vi "Manuel Olcum ile Excele Atma.vi"() -> ()   [LabVIEW 2014]
panel:
  in  "ok":bool
  in  "Kelvin Yk-1":dbl format="%.5p"
  in  "Kelvin Yk":dbl format="%.5p"
  in  "Wagner Yk-1":dbl format="%.5p"
  in  "Wagner Yk":dbl format="%.5p"
  in  "1R Yk-1":dbl format="%.5p"
  in  "1R Yk":dbl format="%.5p"
  in  "10R Yk-1":dbl format="%.5p"
  in  "10R Yk":dbl format="%.5p"
  in  "Ana Denge Yk-1":dbl format="%.5p"
  in  "Ana Denge Yk":dbl format="%.5p"
  in  "Cp 1R":dbl format="%_1e"
  in  "Cp 10R":dbl format="%_1e"
  in  "Kelvin Y_2":dbl=2e-07 format="%_1e"
  in  "Kelivn Y_1":dbl=1e-06 format="%_1e"
  in  "Kelvin X_2":dbl=2e-07 format="%_1e"
  in  "Kelvin X_1":dbl=1e-06 format="%_1e"
  in  "Wagner Y_2":dbl=2e-05 format="%_1e"
  in  "Wagner Y_1":dbl=5e-05 format="%_1e"
  in  "Wagner X_2":dbl=2e-05 format="%_1e"
  in  "Wagner X_1":dbl=5e-05 format="%_1e"
  in  "1R Y_2":dbl=1e-05 format="%_1e"
  in  "1R Y_1":dbl=2e-05 format="%_1e"
  in  "1R X_2":dbl=1e-05 format="%_1e"
  in  "1R X_1":dbl=2e-05 format="%_1e"
  in  "10R Y_2":dbl=1e-05 format="%_1e"
  in  "10R Y_1":dbl=2e-05 format="%_1e"
  in  "10R X_2":dbl=1e-05 format="%_1e"
  in  "10R X_1":dbl=2e-05 format="%_1e"
  in  "AD Y_2":dbl=2e-07 format="%_1e"
  in  "AD Y_1":dbl=1e-06 format="%_1e"
  in  "AD X_2":dbl=2e-07 format="%_1e"
  in  "AD X_1":dbl=1e-06 format="%_1e"
  in  "Direnc 2":dbl format="%_1e"
  in  "Direnc 1":dbl format="%_1e"
  in  "Besleme":dbl=1.0
  in  "Frekans":dbl=1000.0
  in  "Kelvin Faz":dbl format="%.3p"
  in  "Wagner Faz":dbl format="%.3p"
  in  "1R Faz":dbl format="%.3p"
  in  "10R Faz":dbl format="%.3p"
  in  "Ana Denge Faz":dbl format="%.3p"
  in  "Kelvin Xk-1":dbl format="%.5p"
  in  "Kelvin Xk":dbl format="%.5p"
  in  "Wagner Xk-1":dbl format="%.5p"
  in  "Wagner Xk":dbl format="%.5p"
  in  "1R Xk-1":dbl format="%.5p"
  in  "1R Xk":dbl format="%.5p"
  in  "10R Xk-1":dbl format="%.5p"
  in  "10R Xk":dbl format="%.5p"
  in  "Ana Denge Xk-1":dbl format="%.5p"
  in  "Ana Denge Xk":dbl format="%.5p"
  # "Otomatik ölçüm alınabilmesi için gereken değerler"
  # "Ana Denge Ve Kelvin İçin Range Değeri"
  # "5uV"
  # "10R, 1R ve Wagner İçin Range Değeri"
  # "500uV"
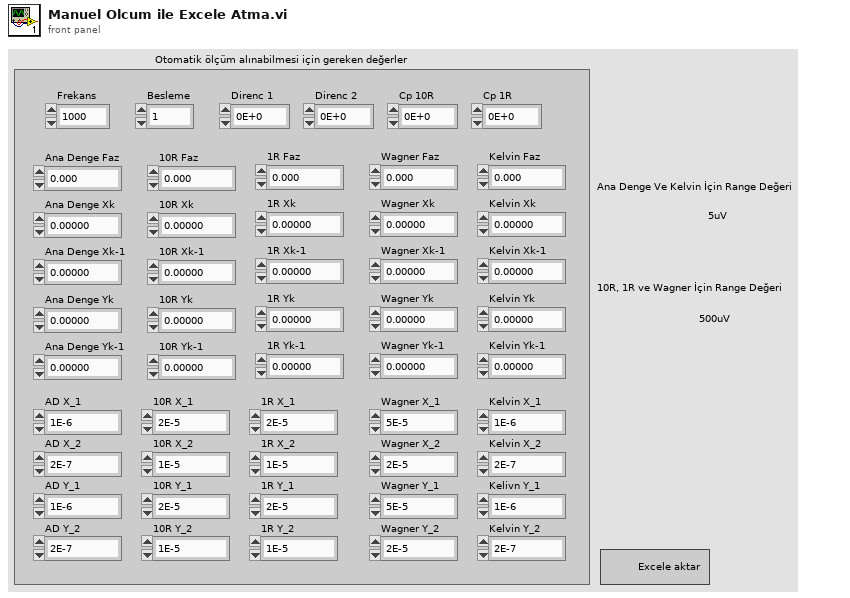
[diagram p1: front panel]
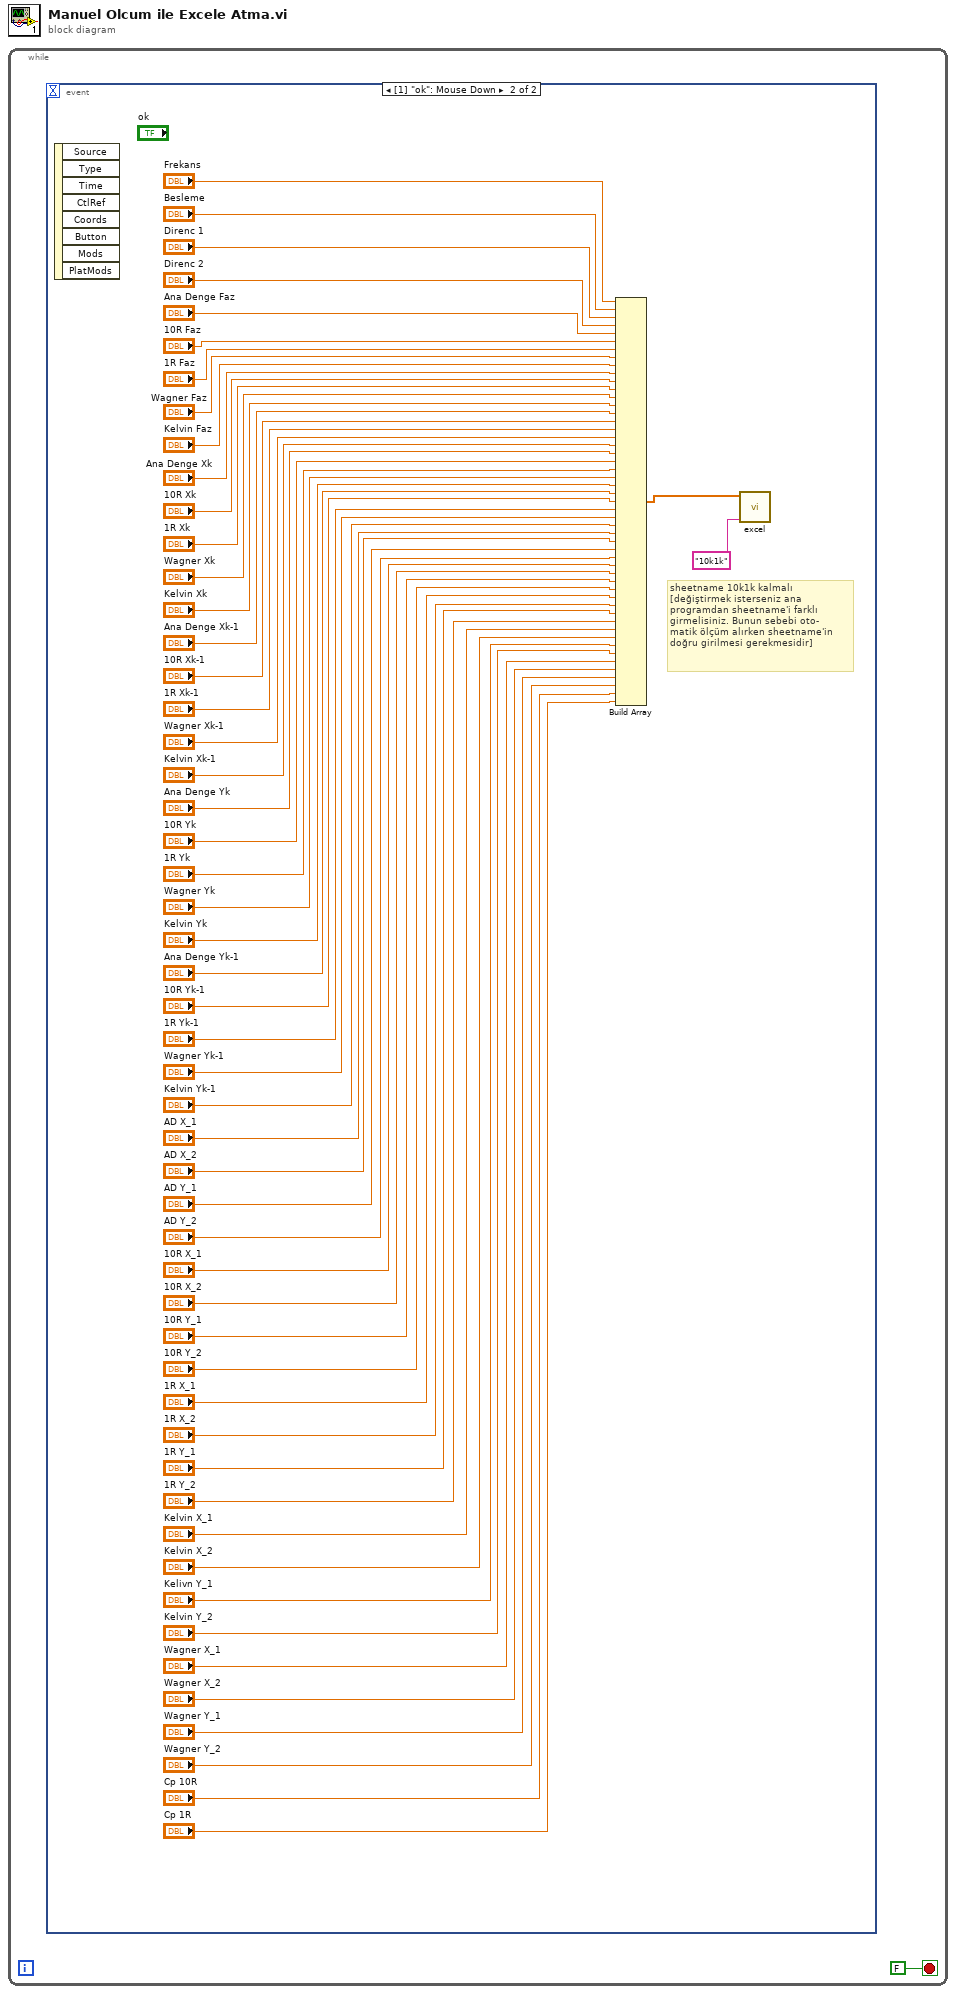
[diagram p0: block diagram]
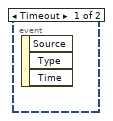
[diagram p2: hidden frame]
diagram:
  n1 = while {
    stop <- FALSE stop-if-true
    n2 = event shown="[1] \"ok\": Mouse Down" {
      selector: _ -> [_ _]
      dyn-events: _ -> [_ _]
      timeout: _ -> [_ _]
      event Timeout {
        n3 = event-data() -> ()  [unwired: 1 in, 3 out]
      }
      event "ok": Mouse Down {
        # "sheetname 10k1k kalmalı\n[değiştirmek isterseniz ana \nprogramdan sheetname'i farklı\ngirmelisiniz. Bunun sebebi oto-\nmatik ölçüm alırken sheetname'in \ndoğru girilmesi gerekmesidir]"
        n4 = event-data() -> ()  [unwired: 1 in, 8 out]
        n5 = Build Array("Frekans", "Besleme", "Direnc 1", "Direnc 2", "Ana Denge Faz", "10R Faz", "1R Faz", "Wagner Faz", "Kelvin Faz", "Ana Denge Xk", "10R Xk", "1R Xk", "Wagner Xk", "Kelvin Xk", "Ana Denge Xk-1", "10R Xk-1", "1R Xk-1", "Wagner Xk-1", "Kelvin Xk-1", "Ana Denge Yk", "10R Yk", "1R Yk", "Wagner Yk", "Kelvin Yk", "Ana Denge Yk-1", "10R Yk-1", "1R Yk-1", "Wagner Yk-1", "Kelvin Yk-1", "AD X_1", "AD X_2", "AD Y_1", "AD Y_2", "10R X_1", "10R X_2", "10R Y_1", "10R Y_2", "1R X_1", "1R X_2", "1R Y_1", "1R Y_2", "Kelvin X_1", "Kelvin X_2", "Kelivn Y_1", "Kelvin Y_2", "Wagner X_1", "Wagner X_2", "Wagner Y_1", "Wagner Y_2", "Cp 10R", "Cp 1R") -> (w2:dbl[])
        n6 = call "excel.vi"("1d array"=w2, "Sheet name"="10k1k") -> ()  [unwired: 9 in]
      }
    }
  }
